vi "Get State.vi"(8 "error in (no error)":errorcluster, 11 "Pulse Controller in":refnum<class "Pulse Recorder.lvclass">) -> (0 "error out":errorcluster, 1 "Result ready":bool, 2 "Armed":bool, 3 "Pulse Controller out":refnum<class "Pulse Recorder.lvclass">)   [LabVIEW 2016, in "Pulse Recorder.lvclass"]
uses:
  Pulse Recorder.lvclass
  D:/github/Measure_core/Measure Object/Measure Object.lvclass
  Pulse Recorder.lvclass/Pulse Recorder.ctl
  Measure Object/Measure Object.lvclass/Measure Object.ctl
  Measure Object Messages/Self-Addressed Msg/Self-addressed Msg.lvclass/Self-addressed Msg.ctl
  Controllers/Pulse Controller Messages/Armed Response Msg/Armed Response Msg.lvclass/Armed Response Msg.ctl
  <vilib>/ActorFramework/Message Enqueuer/Message Enqueuer.lvclass/Message Enqueuer.ctl
  Measure Object/Read Name.vi
  Measure Object/Read Reply to.vi
  Measure Object Messages/Self-Addressed Msg/Read Return Enqueuer.vi
  <vilib>/ActorFramework/Message Enqueuer/Enqueue.vi
  Measure Object Messages/Result Reply Msg/Result Reply Msg.lvclass
  D:/github/Measure_core/Measure Object Messages/Self-Addressed Msg/Self-addressed Msg.lvclass
  Controllers/Pulse Controller Messages/Armed Response Msg/Armed Response Msg.lvclass
  D:/Program Files/National Instruments/LabVIEW 2016/vi.lib/ActorFramework/Message/Message.lvclass
  <vilib>/ActorFramework/Message Priority Queue/Priority Enqueue.vi
  <vilib>/ActorFramework/Message Enqueuer/Message Enqueuer.lvclass
  Instrument Recorders/Instrument Recorder/Instrument Recorder.lvclass
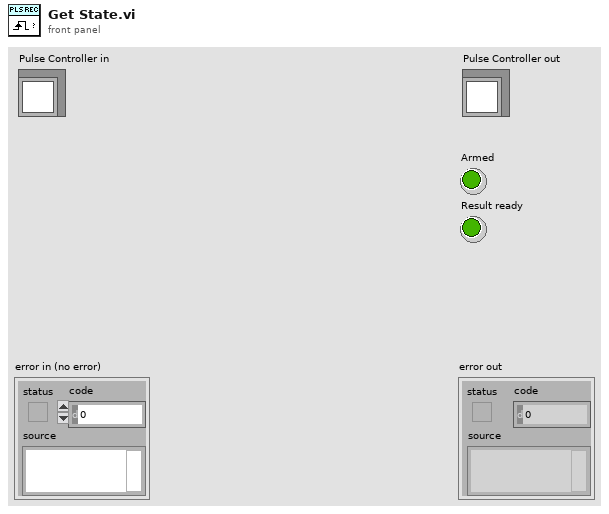
[diagram p1: front panel]
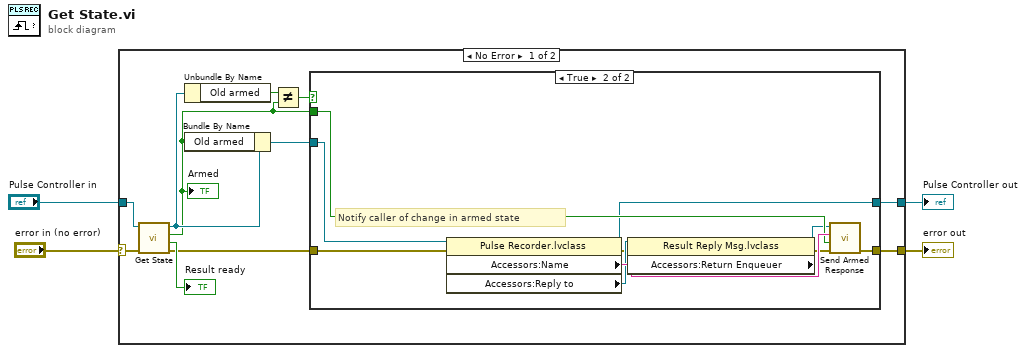
[diagram p0: block diagram]
diagram:
  n1 = case shown="No Error" "error in (no error)" {
    selector: "error in (no error)" -> [w11 w29]
    tunnel: [w12 w29] -> w3
    tunnel: [w8 w28] -> w1
    tunnel: "Pulse Controller in" -> [w10 w28]
    frame No Error {
      n2 = call-parent "Get State.vi"("error in (no error)"=w11, "Pulse Controller in"=w10) -> ("error out"=w5:errorcluster, "Result ready"=→"Result ready":bool, "Armed"=w7:bool, "Pulse Controller out"=w9:refnum<class "Pulse Recorder.lvclass">)  [unwired: 6 in]
      "Armed" <- w7
      n3 = Unbundle By Name(w9) -> ("Old armed"=w15:bool)
      n4 = Bundle By Name(cluster=w9, "Old armed"=w7) -> (w13:refnum<class "Pulse Recorder.lvclass">)
      n5 = Not Equal?(x=w15, y=w7) -> (x != y?=w14:bool)
      n6 = case shown="True" w14 {
        tunnel: w13 -> [w16 w27]
        tunnel: w5 -> [w17 w18]
        tunnel: [w17 w25] -> w12
        tunnel: w7 -> [_ w24]
        tunnel: [w16 w23] -> w8
        frame False {
        }
        frame True {
          # "Notify caller of change in armed state"
          n7 = property class="Pulse Recorder.lvclass"(reference=w27, error in=w18) -> (reference out=w23:refnum<class "Pulse Recorder.lvclass">, error out=w19:errorcluster, "Accessors:Name"=w26:string, "Accessors:Reply to"=w22:refnum<class "Result Reply Msg.lvclass">)
          n8 = property class="Result Reply Msg.lvclass"(reference=w22, error in=w19) -> (error out=w20:errorcluster, "Accessors:Return Enqueuer"=w21:refnum<class "Message Enqueuer.lvclass">)  [unwired: 1 out]
          n9 = call "Send Armed Response.vi"("error in (no error)"=w20, "Armed"=w24, "Sender"=w26, "Message Enqueuer"=w21) -> ("error out"=w25:errorcluster)  [unwired: 6 in, 1 out]
        }
      }
    }
    frame Error {
    }
  }
  "error out" <- w3
  "Pulse Controller out" <- w1
